vi "Untitled 1.vi"() -> ()   [LabVIEW 2015, in "E2E Tag Exchange editor node.lvclass"]
uses:
  E2E Tag Exchange editor node.lvclass
  Pairing Tab References.ctl
panel:
  in  "Pairing Tab Refs":T1
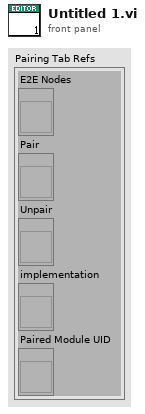
[diagram p1: front panel]
types:
  T1 = typedef "E2E Tag Exchange editor node.lvclass/Pairing Tab References.ctl" = cluster{"E2E Nodes":refnum<vi>, "Pair":refnum<vi>, "Unpair":refnum<vi>, "implementation":refnum<vi>, "Paired Module UID":refnum<vi>}
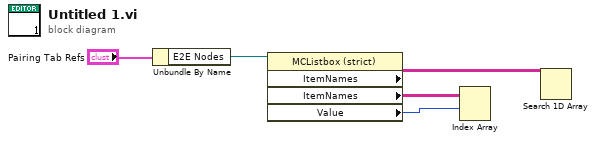
[diagram p0: block diagram]
diagram:
  n1 = Unbundle By Name("Pairing Tab Refs") -> ("E2E Nodes"=w4:refnum<vi>)
  n2 = property class="MCListbox (strict)"(reference=w4) -> ("ItemNames"=w1:string[][], "ItemNames"=w3:string[][], "Value"=w2:i32)  [unwired: 1 in, 2 out]
  n3 = Index Array(array=w3, index (row)=w2) -> ()  [unwired: 1 in, 1 out]
  n4 = Search 1D Array(1D array=w1) -> ()  [unwired: 2 in, 1 out]
